vi "Handle Error.vi"(8 "error in (no error)":errorcluster, 11 "Island Watch in":refnum<class "Island Watch.lvclass">) -> (0 "error out":errorcluster, 2 "stop actor?":bool=TRUE, 3 "Island Watch out":refnum<class "Island Watch.lvclass">)   [LabVIEW 2015, in "Island Watch Actor.lvlib" / "Island Watch.lvclass"]
doc: "(<B>Filename</B>: Actor Framework.lvlib:Actor.lvclass:Handle Error.vi)\n\nDefines how the actor handles an error that occurred while processing a message. By default, this method does nothing except stop the actor."
uses:
  Island Watch.lvclass
  <vilib>/ActorFramework/Actor/Actor.lvclass
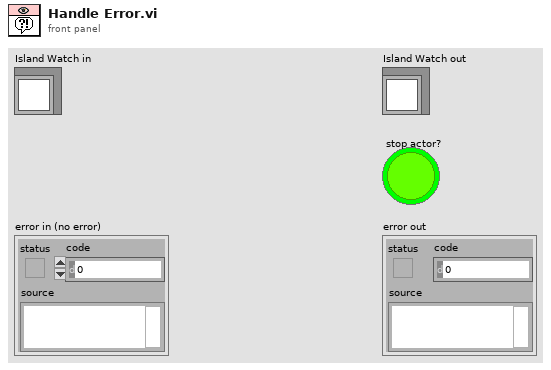
[diagram p1: front panel]
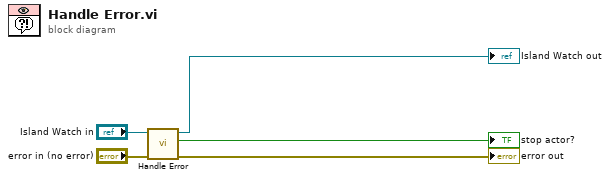
[diagram p0: block diagram]
diagram:
  n1 = call-parent "Handle Error.vi"("error in (no error)"="error in (no error)", "Actor in"="Island Watch in") -> ("error out"=→"error out":errorcluster, "stop actor?"=→"stop actor?":bool, "Actor out"=→"Island Watch out":refnum<class "Island Watch.lvclass">)  [unwired: 7 in]
